vi "Dot.vi"(8 "error in":errorcluster, 10 "Vec3d in 2":refnum<class "Vec3d.lvclass">, 11 "Vec3d in 1":refnum<class "Vec3d.lvclass">) -> (0 "error out":errorcluster, 2 "Dot Product":dbl)   [LabVIEW 2017, in "Vec3d.lvclass"]
uses:
  Vec3d.lvclass
  Vec3d.lvclass/Vec3d.ctl
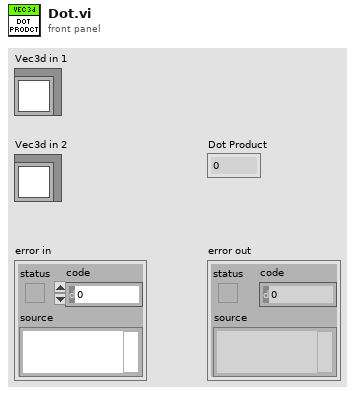
[diagram p1: front panel]
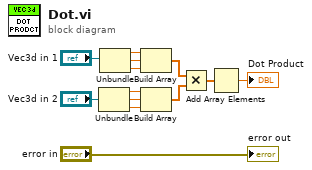
[diagram p0: block diagram]
diagram:
  n1 = Unbundle("Vec3d in 2") -> (w7:dbl, w6:dbl, w5:dbl)
  n2 = Unbundle("Vec3d in 1") -> (w10:dbl, w9:dbl, w8:dbl)
  n3 = Build Array(w10, w9, w8) -> (w4:dbl[])
  n4 = Build Array(w7, w6, w5) -> (w3:dbl[])
  n5 = Multiply(x=w4, y=w3) -> (x*y=w2:dbl[])
  n6 = Add Array Elements(numeric array=w2) -> (sum=→"Dot Product":dbl)
  "error out" <- "error in"
